vi "2012_01_17 Quality Crunch.vi"(8 "error in (no error)":errorcluster, 9 "data":waveform(dbl)[](array[waveform]), 10 "Elapsed Time (s)":dbl, 11 "Motor In":T1 {"No Load Torque" format="%.3f"; "Stall Torque" format="%.3f"; "ESC Efficiency" format="%#_3g%%"; "Supply Power (W)" format="%.3f"; "Mechanical Power (W)" format="%.3f"; "Motor Efficiency" format="%#_3g%%"; "Electrical Power (W)" format="%.3f"; "Torque (mNm)" format="%.3f"; "Elapsed Time" format="%<%H:%M:%S>t"; "Supply (V)" format="%.2f"; "RPM" scale=0.0..60000.0}) -> (0 "error out":errorcluster, 2 "Dynamic Data Type":dynamicdata(waveform), 3 "Motor Out":T1={"Write"=FALSE, "Fail"=FALSE, "RPM"=0, "Motor"=enum."Maxon EC6 6V", "ESC"=enum."Phoenix", "Supply (V)"=0.0, "Test ID and Serial #"="", "Comments"="", "Elapsed Time"=0.0, "Counter"=0.0, "Torque (mNm)"=0.0, "Electrical Power (W)"=0.0, "Motor Efficiency"=0.0, "Mechanical Power (W)"=0.0, "Supply Power (W)"=0.0, "ESC Efficiency"=0.0, "No Load Speed"=0, "Stall Torque"=0.0, "Speed/Torque Gradient"=0, "Calcul"=FALSE, "Clear"=FALSE, "No Load Torque"=0.0} {"No Load Torque" format="%.3f"; "Stall Torque" format="%.3f"; "ESC Efficiency" format="%#_3g%%"; "Supply Power (W)" format="%.3f"; "Mechanical Power (W)" format="%.3f"; "Motor Efficiency" format="%#_3g%%"; "Electrical Power (W)" format="%.3f"; "Torque (mNm)" format="%.3f"; "Elapsed Time" format="%<%H:%M:%S>t"; "Supply (V)" format="%.2f"; "RPM" scale=0.0..60000.0})   [LabVIEW 2013]
uses:
  Quality Type Def.ctl
  <vilib>/measure/matone.llb/Extract Single Tone Information 1 Chan.vi
  <vilib>/measure/madcrms.llb/Basic Averaged DC-RMS for 1 Chan.vi
  <vilib>/express/express arith-compare/Formula/XNode/ExpressFormulaBlockNode.xnode
  <vilib>/measure/NI_MAPro.lvlib
panel:
  # "Fail"
  # "Fail"
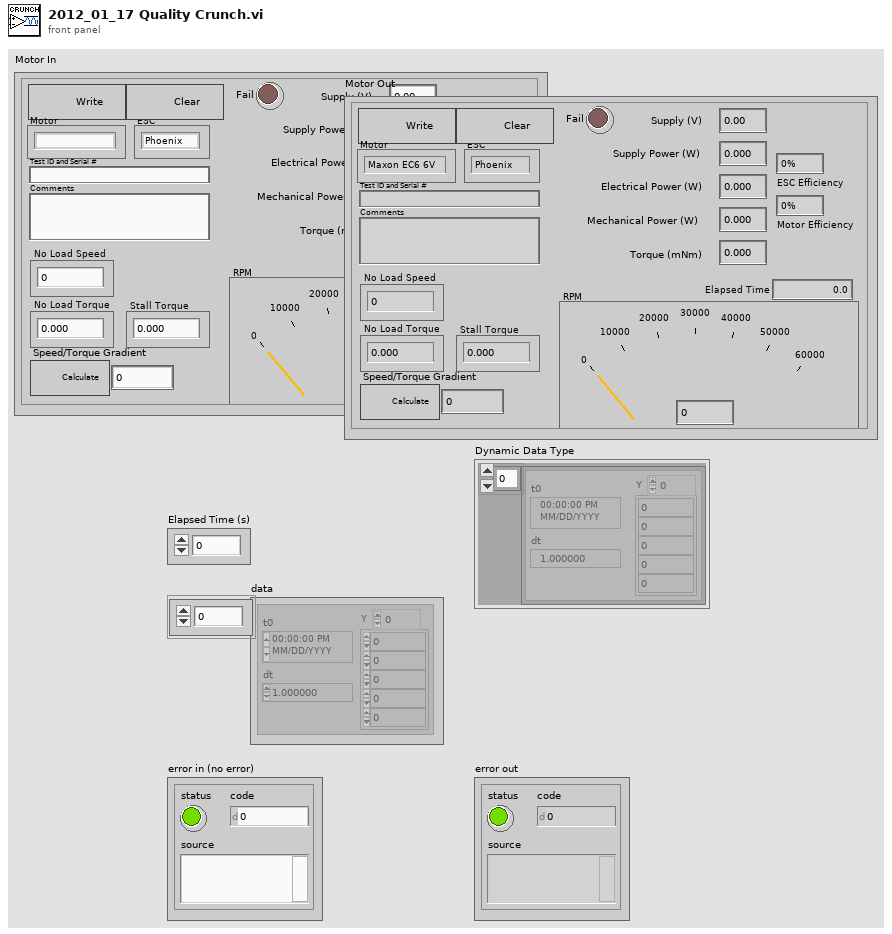
[diagram p1: front panel]
types:
  T1 = typedef "Quality Type Def.ctl" = cluster{"Write":bool, "Fail":bool, "RPM":u64, "Motor":enum16{"", "Maxon EC6 6V", "Maxon EC4 6V", "FH 0620 6V", "FH 0620 12V", "FH 0427 6V K2540"}, "ESC":enum16{"Phoenix", "Maxon", "FH 1801"}, "Supply (V)":dbl, "Test ID and Serial #":string, "Comments":string, "Elapsed Time":dbl, "Counter":dbl, "Torque (mNm)":dbl, "Electrical Power (W)":dbl, "Motor Efficiency":dbl, "Mechanical Power (W)":dbl, "Supply Power (W)":dbl, "ESC Efficiency":dbl, "No Load Speed":u32, "Stall Torque":dbl, "Speed/Torque Gradient":u32, "Calcul":bool, "Clear":bool, "No Load Torque":dbl}
  T2 = enum16{"", "Maxon EC6 6V", "Maxon EC4 6V", "FH 0620 6V", "FH 0620 12V", "FH 0427 6V K2540"}
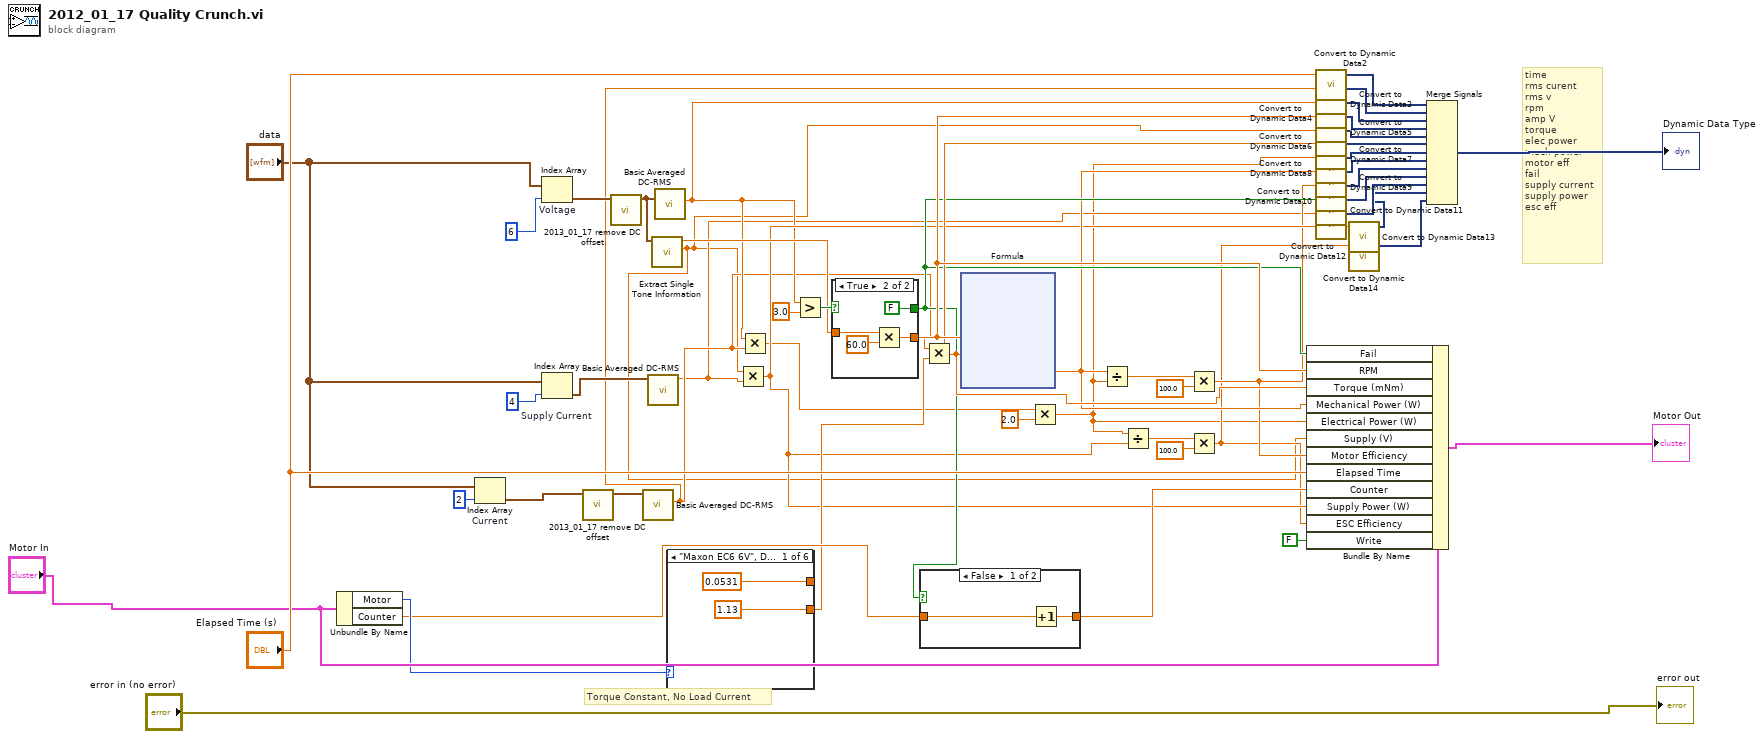
[diagram p0: block diagram]
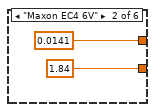
[diagram p3: hidden frame]
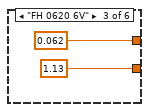
[diagram p4: hidden frame]
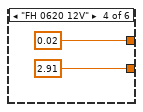
[diagram p5: hidden frame]
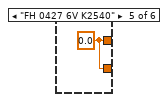
[diagram p6: hidden frame]
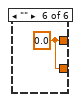
[diagram p7: hidden frame]
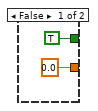
[diagram p8: hidden frame]
diagram:
  # "time\nrms curent\nrms v\nrpm\namp V\ntorque\nelec power\nmech power\nmotor eff\nfail\nsupply current\nsupply power\nesc eff"
  # "Torque Constant, No Load Current"
  n1 = Unbundle By Name("Motor In") -> ("Motor"=w44:T2, "Counter"=w43:dbl)
  n2 = Index Array "Current"(array="data", index=2) -> (element=w27:waveform(dbl))
  n3 = Index Array "Voltage"(array="data", index=6 ("y")) -> (element=w25:waveform(dbl))
  n4 = Index Array "Supply Current"(array="data", index=4) -> (element=w22:waveform(dbl))
  n5 = call "2013_01_17 remove DC offset.vi"("Waveform in"=w27) -> ("Waveform out"=w26:waveform(dbl))  [unwired: 10 in]
  n6 = call "2013_01_17 remove DC offset.vi"("Waveform in"=w25) -> ("Waveform out"=w24:waveform(dbl))  [unwired: 10 in]
  n7 = call-poly <vilib>:"Basic Averaged DC-RMS.vi"("signal in"=w26) -> ("RMS value"=w9:dbl)  [unwired: 7 in, 3 out]
  n8 = call-poly <vilib>:"Basic Averaged DC-RMS.vi"("signal in"=w22) -> ("DC value"=w6:dbl)  [unwired: 7 in, 3 out]
  n9 = call-poly <vilib>:"Extract Single Tone Information.vi"("time signal in"=w24) -> ("detected amplitude"=w5:dbl, "detected frequency"=w45:dbl)  [unwired: 5 in, 4 out]
  n10 = call-poly <vilib>:"Basic Averaged DC-RMS.vi"("signal in"=w24) -> ("RMS value"=w10:dbl)  [unwired: 7 in, 3 out]
  n11 = case shown="\"Maxon EC6 6V\", Default" w44 {
    tunnel: [1.13 1.84 1.13 2.91 w62 w63] -> w21
    tunnel: [0.0531 0.0141 0.062 0.02 w62 w63] -> _
    frame "Maxon EC6 6V", Default {
    }
    frame "Maxon EC4 6V" {
    }
    frame "FH 0620 6V" {
    }
    frame "FH 0620 12V" {
    }
    frame "FH 0427 6V K2540" {
      w62 = 0.0
    }
    frame "" {
      w63 = 0.0
    }
  }
  n12 = Multiply(x=w5, y=w6) -> (x*y=w17:dbl)
  n13 = Multiply(x=w10, y=w9) -> (x*y=w4:dbl)
  n14 = Greater?(x=w10, y=3.0) -> (0:w47:bool)
  n15 = case shown="True" w47 {
    tunnel: [0.0 ("y") w69] -> w42
    tunnel: w45 -> [_ w67]
    tunnel: [TRUE FALSE] -> w29
    frame False {
    }
    frame True {
      n16 = Multiply(x=w67, y=60.0) -> (x*y=w69:dbl)
    }
  }
  n17 = case shown="False" w29 {
    tunnel: w43 -> [w71 w72]
    tunnel: [w70 w72] -> w40
    frame False {
      n18 = Increment(x=w71) -> (x+1=w70:dbl)
    }
    frame True {
    }
  }
  n19 = Multiply(x=w9, y=w21) -> (x*y=w41:dbl)
  n20 = xnode "Formula"("RPM"=w42, "Torque"=w41) -> ("Result"=w18:dbl)  [unwired: 1 in, 1 out]
  n21 = Multiply(x=w4, y=2.0) -> (x*y=w2:dbl)
  n22 = Divide(x=w18, y=w2) -> (x/y=w14:dbl)
  n23 = Divide(x=w2, y=w17) -> (x/y=w12:dbl)
  n24 = Multiply(x=w14, y=100.0) -> (x*y=w13:dbl)
  n25 = Multiply(x=w12, y=100.0) -> (x*y=w11:dbl)
  n26 = Bundle By Name(cluster="Motor In", "Fail"=w29, "RPM"=w42, "Torque (mNm)"=w41, "Mechanical Power (W)"=w18, "Electrical Power (W)"=w2, "Supply (V)"=w5, "Motor Efficiency"=w13, "Elapsed Time"="Elapsed Time (s)", "Counter"=w40, "Supply Power (W)"=w17, "ESC Efficiency"=w11, "Write"=FALSE) -> (→"Motor Out":T1)
  n27 = call "Convert to Dynamic Data2"("Double"="Elapsed Time (s)") -> ("Dynamic Data Type"=w39:dynamicdata)  [unwired: 3 in]
  n28 = call "Convert to Dynamic Data3"("Double"=w9) -> ("Dynamic Data Type"=w38:dynamicdata)  [unwired: 3 in]
  n29 = call "Convert to Dynamic Data4"("Double"=w10) -> ("Dynamic Data Type"=w37:dynamicdata)  [unwired: 3 in]
  n30 = call "Convert to Dynamic Data5"("Double"=w42) -> ("Dynamic Data Type"=w36:dynamicdata)  [unwired: 3 in]
  n31 = call "Convert to Dynamic Data6"("Double"=w5) -> ("Dynamic Data Type"=w35:dynamicdata)  [unwired: 3 in]
  n32 = call "Convert to Dynamic Data7"("Double"=w41) -> ("Dynamic Data Type"=w34:dynamicdata)  [unwired: 3 in]
  n33 = call "Convert to Dynamic Data8"("Double"=w2) -> ("Dynamic Data Type"=w33:dynamicdata)  [unwired: 3 in]
  n34 = call "Convert to Dynamic Data9"("Double"=w18) -> ("Dynamic Data Type"=w32:dynamicdata)  [unwired: 3 in]
  n35 = call "Convert to Dynamic Data10"("Double"=w13) -> ("Dynamic Data Type"=w31:dynamicdata)  [unwired: 3 in]
  n36 = call "Convert to Dynamic Data11"("Boolean"=w29) -> ("Dynamic Data Type"=w30:dynamicdata)  [unwired: 3 in]
  n37 = call "Convert to Dynamic Data12"("Double"=w6) -> ("Dynamic Data Type"=w28:dynamicdata)  [unwired: 3 in]
  n38 = call "Convert to Dynamic Data13"("Double"=w17) -> ("Dynamic Data Type"=w20:dynamicdata)  [unwired: 3 in]
  n39 = call "Convert to Dynamic Data14"("Double"=w11) -> ("Dynamic Data Type"=w19:dynamicdata)  [unwired: 3 in]
  n40 = Merge Signals(w39, w38, w37, w36, w35, w34, w33, w32, w31, w30, w28, w20, w19) -> (→"Dynamic Data Type":dynamicdata)
  "error out" <- "error in (no error)"
